vi "ep_Check Frequency Domain Parameters.vi"(0 "spectra in":T2(array[cluster]), 5 "gains":dbl[][][](array[numeric]), 7 "phase delays [deg]":dbl[][][](array[numeric]), 11 "error in (no error)":errorcluster, 12 "frequencies to calibrate [Hz]":dbl[](array[numeric]), 13 "ranges to calibrate [%]":dbl[](array[numeric]), 14 "actual ranges [%]":dbl[](array[numeric])) -> (15 "error out":errorcluster)   [LabVIEW 2014, in "NI_EP_Power Quality.lvlib"]
uses:
  <vilib>/addons/Electrical Power/PQ/NI_EP_Power Quality.lvlib
  <vilib>/addons/Electrical Power/PQ/Common/Controls/ep_AI Data Channel.ctl
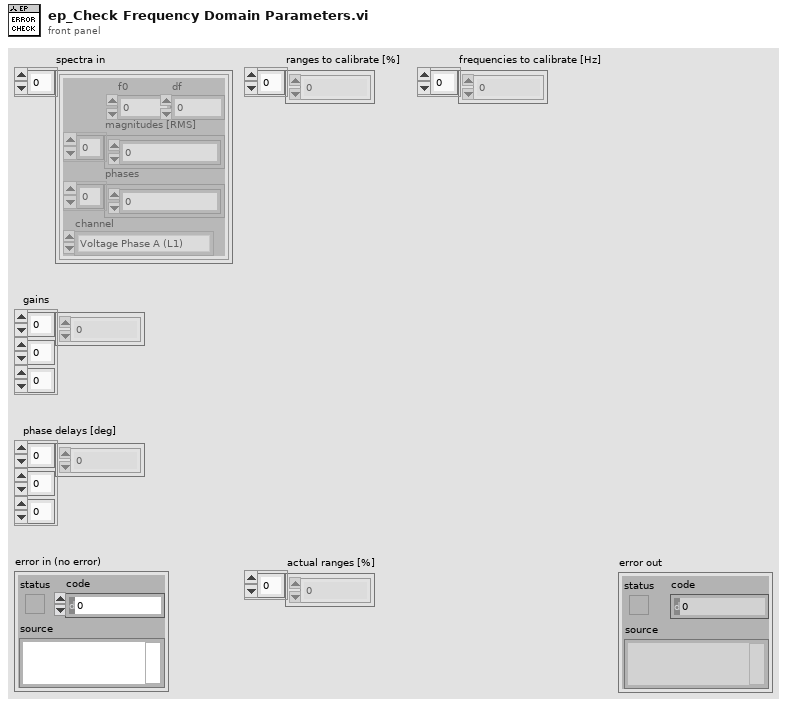
[diagram p1: front panel]
types:
  T1 = typedef "NI_EP_Power Quality.lvlib/ep_AI Data Channel.ctl" = enum16{"Voltage Phase A (L1)", "Voltage Phase B (L2)", "Voltage Phase C (L3)", "Voltage Phase N (Neutral)", "Current Phase A (L1)", "Current Phase B (L2)", "Current Phase C (L3)", "Current Phase N (Neutral)"}
  T2 = cluster{"f0":dbl, "df":dbl, "magnitudes [RMS]":dbl[], "phases":dbl[], "channel":T1}[]
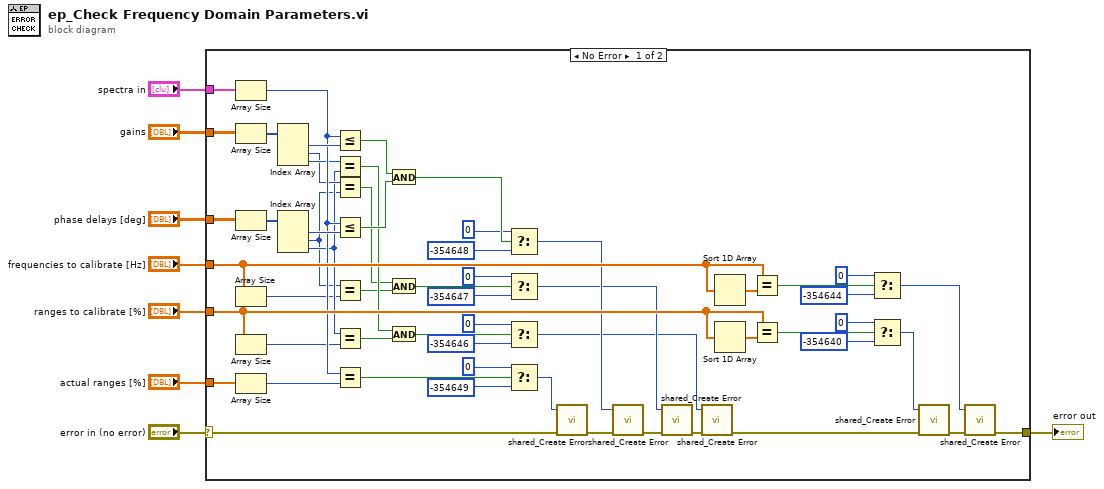
[diagram p0: block diagram]
diagram:
  n1 = case shown="No Error" "error in (no error)" {
    selector: "error in (no error)" -> [w10 w66]
    tunnel: "frequencies to calibrate [Hz]" -> [w57 _]
    tunnel: "ranges to calibrate [%]" -> [w56 _]
    tunnel: "actual ranges [%]" -> [w55 _]
    tunnel: "phase delays [deg]" -> [w54 _]
    tunnel: "spectra in" -> [w52 _]
    tunnel: "gains" -> [w38 _]
    tunnel: [w11 w66] -> w2
    frame No Error {
      n2 = Array Size(array=w52) -> (size(s)=w50:i32)
      n3 = Array Size(array=w38) -> (size(s)=w53:i32[])
      n4 = Array Size(array=w54) -> (size(s)=w64:i32[])
      n5 = Array Size(array=w57) -> (size(s)=w36:i32)
      n6 = Array Size(array=w56) -> (size(s)=w35:i32)
      n7 = Array Size(array=w55) -> (size(s)=w65:i32)
      n8 = Index Array(array=w53) -> (element #1=w51:i32, element #2=w42:i32, element #3=w43:i32)  [unwired: 3 in]
      n9 = Index Array(array=w64) -> (element #1=w63:i32, element #2=w9:i32, element #3=w37:i32)  [unwired: 3 in]
      n10 = Less Or Equal?(x=w50, y=w51) -> (x <= y?=w49:bool)
      n11 = Equal?(x=w43, y=w37) -> (x = y?=w46:bool)
      n12 = Equal?(x=w42, y=w9) -> (x = y?=w39:bool)
      n13 = Less Or Equal?(x=w50, y=w63) -> (x <= y?=w48:bool)
      n14 = Equal?(x=w9, y=w36) -> (x = y?=w41:bool)
      n15 = Equal?(x=w37, y=w35) -> (x = y?=w45:bool)
      n16 = Equal?(x=w50, y=w65) -> (x = y?=w60:bool)
      n17 = And(x=w49, y=w48) -> (x .and. y?=w47:bool)
      n18 = And(x=w39, y=w41) -> (x .and. y?=w40:bool)
      n19 = And(x=w46, y=w45) -> (x .and. y?=w44:bool)
      n20 = Select(t=0 ("error code (0)"), s=w47, f=-354648 ("error code (0)")) -> (s? t:f=w27:i32)
      n21 = Select(t=0 ("error code (0)"), s=w40, f=-354647 ("error code (0)")) -> (s? t:f=w23:i32)
      n22 = Select(t=0 ("error code (0)"), s=w44, f=-354646 ("error code (0)")) -> (s? t:f=w20:i32)
      n23 = Select(t=0 ("error code (0)"), s=w60, f=-354649 ("error code (0)")) -> (s? t:f=w29:i32)
      n24 = call <vilib>:"shared_Create Error.vi"("error in (no error)"=w10, "error code (0)"=w29) -> ("error out"=w26:errorcluster)  [unwired: 9 in]
      n25 = call <vilib>:"shared_Create Error.vi"("error in (no error)"=w26, "error code (0)"=w27) -> ("error out"=w24:errorcluster)  [unwired: 9 in]
      n26 = call <vilib>:"shared_Create Error.vi"("error in (no error)"=w24, "error code (0)"=w23) -> ("error out"=w21:errorcluster)  [unwired: 9 in]
      n27 = call <vilib>:"shared_Create Error.vi"("error in (no error)"=w21, "error code (0)"=w20) -> ("error out"=w15:errorcluster)  [unwired: 9 in]
      n28 = Sort 1D Array(array=w57) -> (sorted array=w58:dbl[])
      n29 = Sort 1D Array(array=w56) -> (sorted array=w62:dbl[])
      n30 = Equal?(x=w57, y=w58) -> (x = y?=w59:bool)
      n31 = Equal?(x=w56, y=w62) -> (x = y?=w61:bool)
      n32 = Select(t=0 ("error code (0)"), s=w59, f=-354644 ("error code (0)")) -> (s? t:f=w12:i32)
      n33 = Select(t=0 ("error code (0)"), s=w61, f=-354640 ("error code (0)")) -> (s? t:f=w16:i32)
      n34 = call <vilib>:"shared_Create Error.vi"("error in (no error)"=w15, "error code (0)"=w16) -> ("error out"=w14:errorcluster)  [unwired: 9 in]
      n35 = call <vilib>:"shared_Create Error.vi"("error in (no error)"=w14, "error code (0)"=w12) -> ("error out"=w11:errorcluster)  [unwired: 9 in]
    }
    frame Error {
    }
  }
  "error out" <- w2
